vi "Read Recording Location.vi"(8 "error in (no error)":errorcluster, 11 "TrialBasedExperiment in":refnum<class "MatlabExperiment.lvclass">) -> (0 "error out":errorcluster, 3 "TrialBasedExperiment out":refnum<class "MatlabExperiment.lvclass">)   [LabVIEW 2014, in "AcquisitionCoreObjects.lvlib" / "MatlabExperiment.lvclass"]
uses:
  MatlabExperiment.lvclass
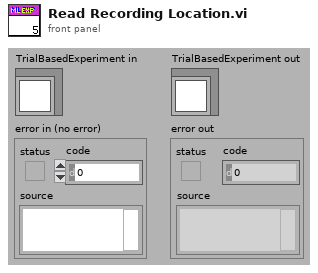
[diagram p1: front panel]
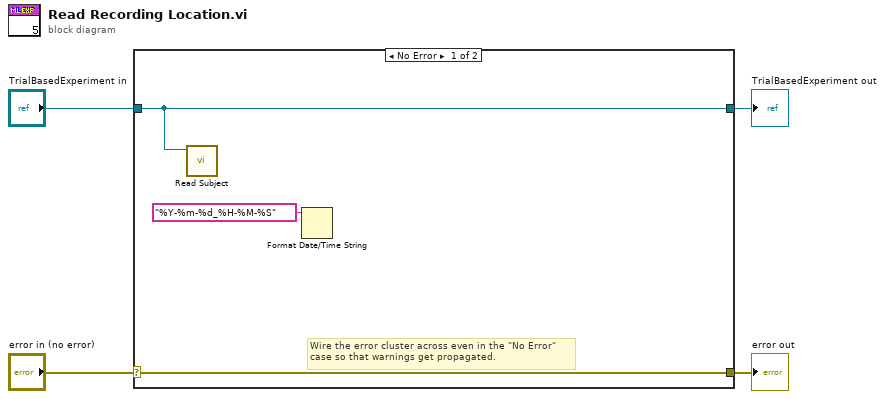
[diagram p0: block diagram]
diagram:
  n1 = case shown="No Error" "error in (no error)" {
    selector: "error in (no error)" -> [w7 w9]
    tunnel: [w7 w9] -> w3
    tunnel: [w6 w8] -> w1
    tunnel: "TrialBasedExperiment in" -> [w6 w8]
    frame No Error {
      # "Wire the error cluster across even in the \"No Error\"\ncase so that warnings get propagated."
      n2 = call-dynamic "Read Subject.vi"("TrialBasedExperiment in"=w6) -> ()  [unwired: 8 in, 3 out]
      n3 = Format Date/Time String(time format string (%c)="%Y-%m-%d_%H-%M-%S") -> ()  [unwired: 3 out]
    }
    frame Error {
    }
  }
  "error out" <- w3
  "TrialBasedExperiment out" <- w1
